vi "CrossTheLineLabview.vi"() -> ()   [LabVIEW 2017]
panel:
  in  "stop":bool
  out "MotorValues 2":dbl
  out "MotorValues":dbl
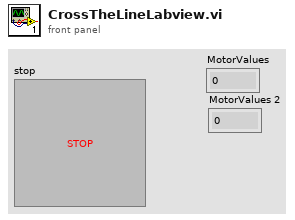
[diagram p1: front panel]
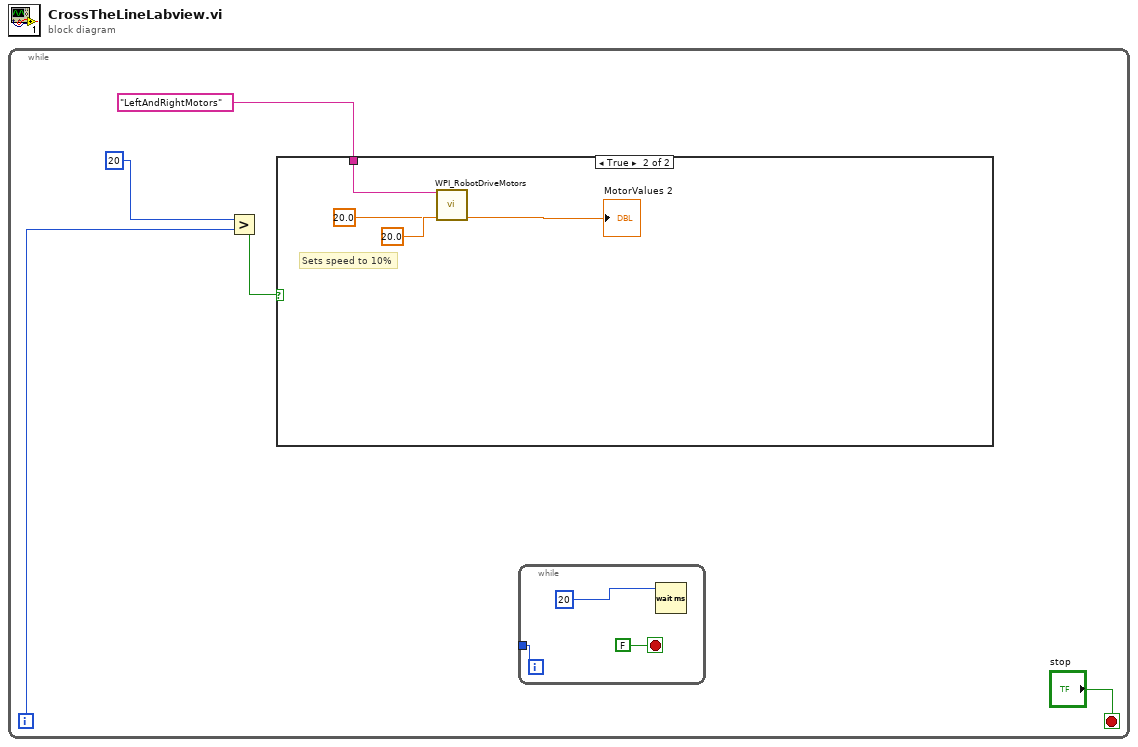
[diagram p0: block diagram]
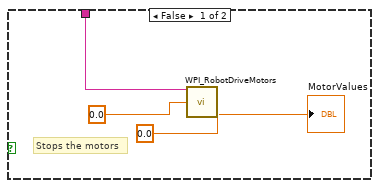
[diagram p2: hidden frame]
diagram:
  n1 = while {
    i -> [w1]
    stop <- "stop" stop-if-true
    n2 = Greater?(x=20, y=w1) -> (0:w5:bool)
    n3 = case shown="True" w5 {
      tunnel: "LeftAndRightMotors" ("RobotDriveDevRef") -> [w7 w11]
      frame False {
        # "Stops the motors"
        n4 = call "WPI_RobotDriveMotors.vi"("RobotDriveDevRef"=w7, "LeftSpeed"=0.0, "RightSpeed"=0.0) -> ("MotorValues"=→"MotorValues":dbl)  [unwired: 11 in, 1 out]
      }
      frame True {
        # "Sets speed to 10%"
        n5 = call "WPI_RobotDriveMotors.vi"("RobotDriveDevRef"=w11, "LeftSpeed"=20.0, "RightSpeed"=20.0) -> ("MotorValues"=→"MotorValues 2":dbl)  [unwired: 11 in, 1 out]
      }
    }
    n6 = while {
      tunnel: [w14] -> _
      i -> [w14]
      stop <- FALSE stop-if-true
      n7 = Wait (ms)(milliseconds to wait=u32 20) -> ()  [unwired: 1 out]
    }
  }
